vi "sg Get Device List.vi"(8 "error in (no error)":errorcluster, 10 "length":i32, 11 "deviceList":i32[](array[numeric])=[0, 0, 0, 0, 0, 0, 0, 0, 0, 0, 0, 0, 0, 0, 0, 0]) -> (0 "error out":errorcluster, 1 "function return":u32(ring), 2 "length out":i32, 3 "deviceList out":i32[](array[numeric]))   [LabVIEW 2014, in "VSG25A.lvlib"]
doc: "SG_API sgStatus sgGetDeviceList(int deviceList[16], int *length);"
uses:
  VSG25A.lvlib
  sg_api.dll
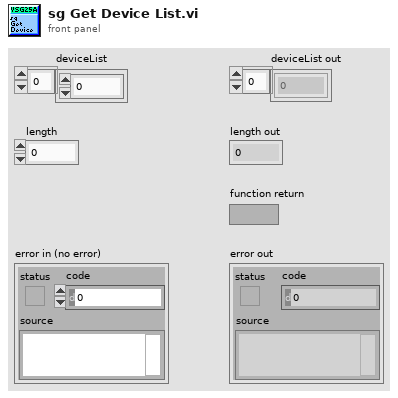
[diagram p1: front panel]
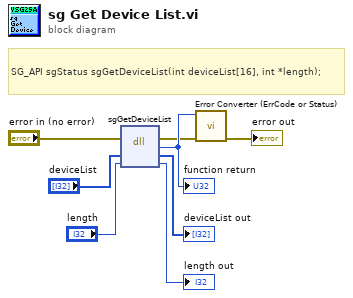
[diagram p0: block diagram]
diagram:
  # "SG_API sgStatus sgGetDeviceList(int deviceList[16], int *length);"
  n1 = dll-call lib="C:/Users/M_LAPTOP/Desktop/Labview/practice/VSG25A/sg_lib/sg_api.*" fn="sgGetDeviceList"(error in="error in (no error)", "deviceList"="deviceList", "length"="length") -> (error out=w2:errorcluster, w8:u32, "deviceList"=→"deviceList out":i32[], "length"=→"length out":i32)  [unwired: 2 in, 1 out]
  "function return" <- w8
  n2 = call "Error Converter (ErrCode or Status).vi"("error in (no error)"=w2, "error code"=w8) -> ("error out"=→"error out":errorcluster)  [unwired: 9 in]
